vi "Place Target On Nearest Visible Object.vi"(0 "Focus and Tracking":T3, 1 "Start Coordinates [pix]":refnum<vi>, 5 "System of Reference Interface":T4, 7 "Calibration":T2, 9 "Target":T1, 11 "error in (no error)":errorcluster) -> (4 "Detected":bool, 15 "error out":errorcluster)   [LabVIEW 2012, in "Targeting Unit.lvlib"]
uses:
  Targeting Unit.lvlib
  <vilib>/Analysis/Matrix/Datatypes/RealMatrix.ctl
  <vilib>/Analysis/Matrix/NI_Matrix.lvlib
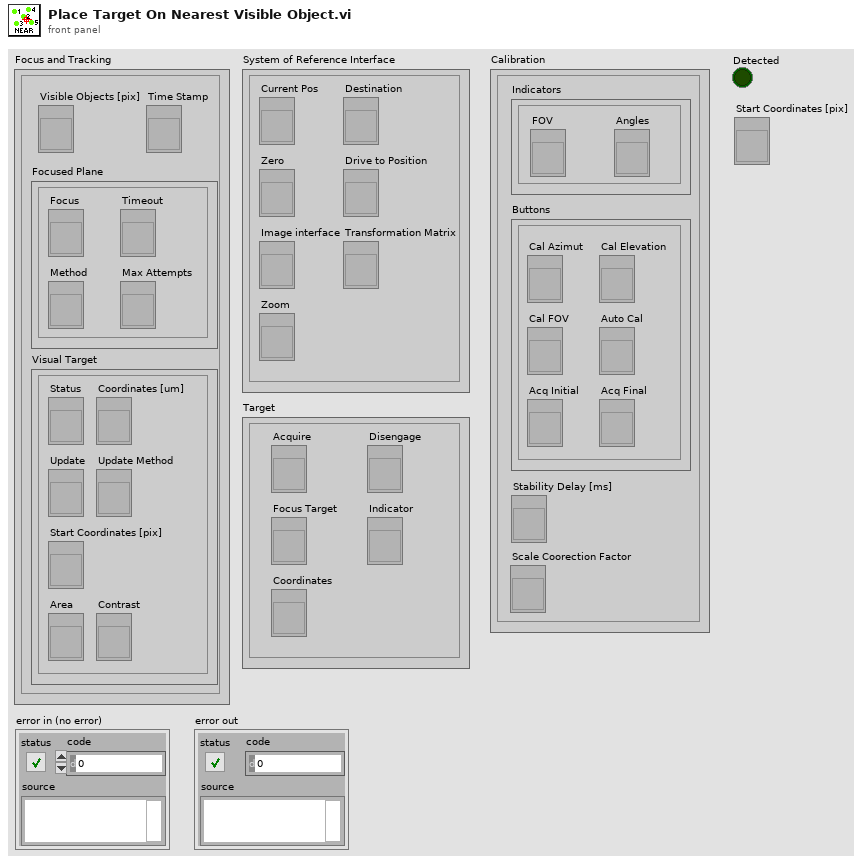
[diagram p1: front panel]
types:
  T1 = cluster{"Coordinates":refnum<vi>, "Acquire":refnum<vi>, "Disengage":refnum<vi>, "Indicator":refnum<vi>, "Focus Target":refnum<vi>}
  T2 = cluster{"Indicators":cluster{"FOV":refnum<vi>, "Angles":refnum<vi>}, "Buttons":cluster{"Cal FOV":refnum<vi>, "Cal Azimut":refnum<vi>, "Cal Elevation":refnum<vi>, "Auto Cal":refnum<vi>, "Acq Initial":refnum<vi>, "Acq Final":refnum<vi>}, "Stability Delay [ms]":refnum<vi>, "Scale Coorection Factor":refnum<vi>}
  T3 = cluster{"Focused Plane":cluster{"Focus":refnum<vi>, "Timeout":refnum<vi>, "Max Attempts":refnum<vi>, "Method":refnum<vi>}, "Time Stamp":refnum<vi>, "Visual Target":cluster{"Coordinates [um]":refnum<vi>, "Status":refnum<vi>, "Update":refnum<vi>, "Update Method":refnum<vi>, "Start Coordinates [pix]":refnum<vi>, "Area":refnum<vi>, "Contrast":refnum<vi>}, "Visible Objects [pix]":refnum<vi>}
  T4 = cluster{"Current Pos":refnum<vi>, "Image interface":refnum<vi>, "Transformation Matrix":refnum<vi>, "Zero":refnum<vi>, "Destination":refnum<vi>, "Drive to Position":refnum<vi>, "Zoom":refnum<vi>}
  T5 = typedef "NI_Matrix.lvlib/RealMatrix.ctl" = dbl[][]
  T6 = cluster{"X [um]":dbl, "Y [um]":dbl, "Z [um]":dbl}
  T7 = cluster{"Area":dbl, "Centre of Mass":cluster{"X":dbl, "Y":dbl}, "Global Rectangle":cluster{"Left":dbl, "Top":dbl, "Right":dbl, "Bottom":dbl}, "Contrast":dbl}[]
  T8 = cluster{"Area":dbl, "Centre of Mass":cluster{"X":dbl, "Y":dbl}, "Global Rectangle":cluster{"Left":dbl, "Top":dbl, "Right":dbl, "Bottom":dbl}, "Contrast":dbl}
  T9 = typedef "ROI Descriptor" = cluster{"Global Rectangle":i32[], "Contours":cluster{"ID":enum32{"External", "Internal"}, "Type":u32, "Coordinates":i32[]}[]}
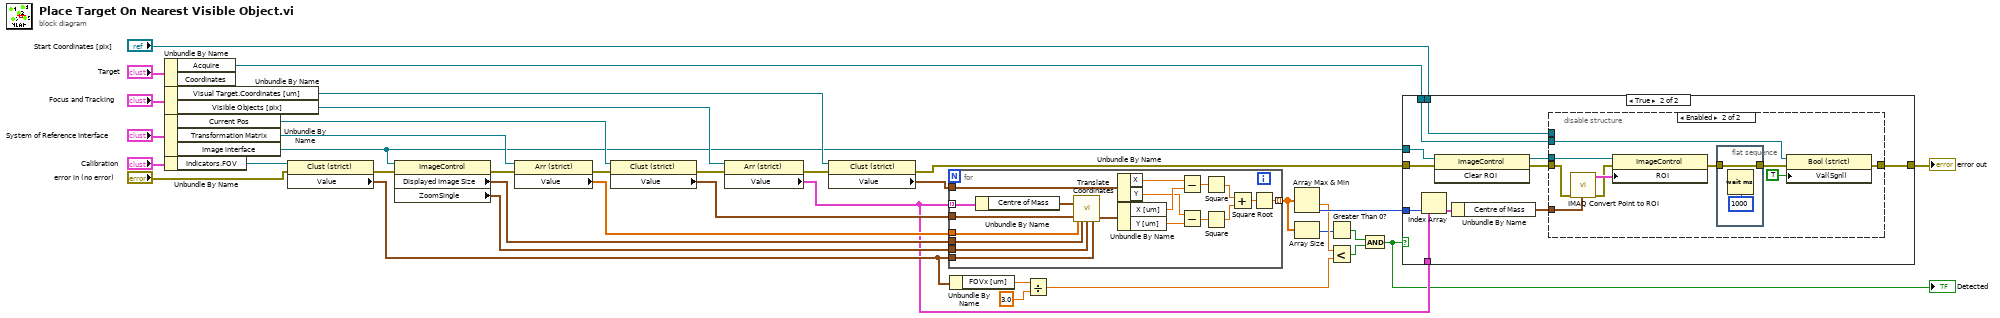
[diagram p0: block diagram]
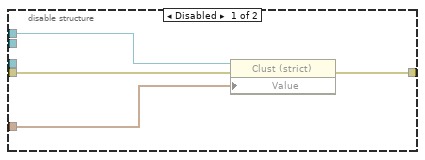
[diagram p3: hidden frame]
diagram:
  n1 = Unbundle By Name("Target") -> ("Acquire"=w7:refnum<vi>)  [unwired: 1 out]
  n2 = Unbundle By Name("Focus and Tracking") -> ("Visual Target.Coordinates [um]"=w23:refnum<vi>, "Visible Objects [pix]"=w35:refnum<vi>)
  n3 = Unbundle By Name("System of Reference Interface") -> ("Current Pos"=w27:refnum<vi>, "Transformation Matrix"=w34:refnum<vi>, "Image interface"=w6:refnum<vi>)
  n4 = Unbundle By Name("Calibration") -> ("Indicators.FOV"=w25:refnum<vi>)
  n5 = property class="Clust (strict)"(reference=w25, error in="error in (no error)") -> (error out=w30:errorcluster, "Value"=w17:cluster{"FOVx [um]":dbl, "FOVy [um]":dbl})  [unwired: 1 out]
  n6 = property class="ImageControl"(reference=w6, error in=w30) -> (error out=w32:errorcluster, "Displayed Image Size"=w28:cluster{"Width":u32, "Height":u32}, "ZoomSingle"=w29:cluster{"X":sgl, "Y":sgl})  [unwired: 1 out]
  n7 = property class="Arr (strict)"(reference=w34, error in=w32) -> (error out=w26:errorcluster, "Value"=w33:T5)  [unwired: 1 out]
  n8 = property class="Clust (strict)"(reference=w27, error in=w26) -> (error out=w12:errorcluster, "Value"=w31:T6)  [unwired: 1 out]
  n9 = property class="Arr (strict)"(reference=w35, error in=w12) -> (error out=w22:errorcluster, "Value"=w10:T7)  [unwired: 1 out]
  n10 = property class="Clust (strict)"(reference=w23, error in=w22) -> (error out=w19:errorcluster, "Value"=w11:cluster{"X":dbl, "Y":dbl, "Z":dbl})  [unwired: 1 out]
  n11 = for {
    tunnel: w10 -> [w56] mode=indexing
    tunnel: w17 -> [w47]
    tunnel: w31 -> [w52]
    tunnel: w33 -> [w51]
    tunnel: w29 -> [w49]
    tunnel: w28 -> [w48]
    tunnel: w11 -> [w46]
    tunnel: [w38] -> w3 mode=indexing
    n12 = Unbundle By Name(w56) -> ("Centre of Mass"=w50:cluster{"X":dbl, "Y":dbl})
    n13 = call "Translate Coordinates.vi"("Transformation Matrix"=w51, "Coordinates [pix]"=w50, "FOV"=w47, "Visualiser Zoom"=w49, "Scope Position"=w52, "Image Area"=w48) -> ("Target Coordinates"=w45:T6)  [unwired: 4 in, 1 out]
    n14 = Unbundle By Name(w46) -> ("X"=w44:dbl, "Y"=w41:dbl)
    n15 = Unbundle By Name(w45) -> ("X [um]"=w43:dbl, "Y [um]"=w42:dbl)
    n16 = Subtract(x=w44, y=w43) -> (x-y=w40:dbl)
    n17 = Subtract(x=w41, y=w42) -> (x-y=w39:dbl)
    n18 = Square(x=w40) -> (x^2=w55:dbl)
    n19 = Square(x=w39) -> (x^2=w54:dbl)
    n20 = Add(x=w55, y=w54) -> (x+y=w53:dbl)
    n21 = Square Root(x=w53) -> (sqrt(x)=w38:dbl)
  }
  n22 = Unbundle By Name(w17) -> ("FOVx [um]"=w16:dbl)
  n23 = Divide(x=w16, y=3.0) -> (x/y=w13:dbl)
  n24 = Array Max & Min(array=w3) -> (min value=w14:dbl, min index (indices)=w20:i32)  [unwired: 2 out]
  n25 = Array Size(array=w3) -> (size(s)=w2:i32)
  n26 = Greater Than 0?(x=w2) -> (x > 0?=w1:bool)
  n27 = Less?(x=w14, y=w13) -> (x < y?=w5:bool)
  n28 = And(x=w1, y=w5) -> (x .and. y?=w4:bool)
  "Detected" <- w4
  n29 = case shown="True" w4 {
    tunnel: w20 -> [_ w65]
    tunnel: w19 -> [w57 w61]
    tunnel: [w57 w68] -> w18
    tunnel: w10 -> [_ w64]
    tunnel: "Start Coordinates [pix]" -> [_ w67]
    tunnel: w7 -> [_ w66]
    tunnel: w6 -> [_ w58]
    frame False {
    }
    frame True {
      n30 = Index Array(array=w64, index=w65) -> (element=w63:T8)
      n31 = invoke class="ImageControl" method="Clear ROI"(reference=w58, error in=w61) -> (reference out=w59:refnum<vi>, error out=w60:errorcluster)  [unwired: 1 in, 1 out]
      n32 = Unbundle By Name(w63) -> ("Centre of Mass"=w62:cluster{"X":dbl, "Y":dbl})
      n33 = disable-structure shown="Enabled" {
        disable-tunnel: w60 -> [w72 w74]
        disable-tunnel: [w71 w80] -> w68
        disable-tunnel: w67 -> [w70 _]
        disable-tunnel: w66 -> [_ w79]
        disable-tunnel: w62 -> [w69 w76]
        disable-tunnel: w59 -> [_ w77]
        frame Disabled {
          n34 = property class="Clust (strict)"(reference=w70, error in=w72, "Value"=w69) -> (error out=w71:errorcluster)  [unwired: 1 out]
        }
        frame Enabled {
          n35 = call "IMAQ Convert Point to ROI"("error in (no error)"=w74, "Point"=w76) -> ("error out"=w73:errorcluster, "ROI Descriptor"=w75:T9)  [unwired: 7 in]
          n36 = property class="ImageControl"(reference=w77, error in=w73, "ROI"=w75) -> (error out=w81:errorcluster)  [unwired: 1 out]
          n37 = flat-sequence {
            tunnel: [w84] -> w82
            tunnel: w81 -> [w84]
            frame #0 {
              n38 = Wait (ms)(milliseconds to wait=u32 1000) -> ()  [unwired: 1 out]
            }
          }
          n39 = property class="Bool (strict)"(reference=w79, error in=w82, "Val(Sgnl)"=TRUE ("Value")) -> (error out=w80:errorcluster)  [unwired: 1 out]
        }
      }
    }
  }
  "error out" <- w18
